vi "Highpass (Host).vi"() -> ()   [LabVIEW 2023]
uses:
  <vilib>/rvi/interface/nirviMethod/nirviMethod.xnode
  <vilib>/rvi/interface/nirviOpenFPGA/nirviOpenFPGA.xnode
  <vilib>/rvi/interface/nirviCloseFPGA/nirviCloseFPGA.xnode
  <vilib>/rvi/errors/niLvFpgaMergeErrorWithErrorCode.vi
  Highpass (FPGA).vi
  FPGA Bitfiles/highpass_FPGATarget_Highpass(FPGA)_je9PWvtYWXA.lvbitx
  <vilib>/userdefined/High Color/nirio_resource_hc.ctl
panel:
  in  "resource name":T1
  out "Filtered Signal":dbl[](graph)
  in  "stop":bool
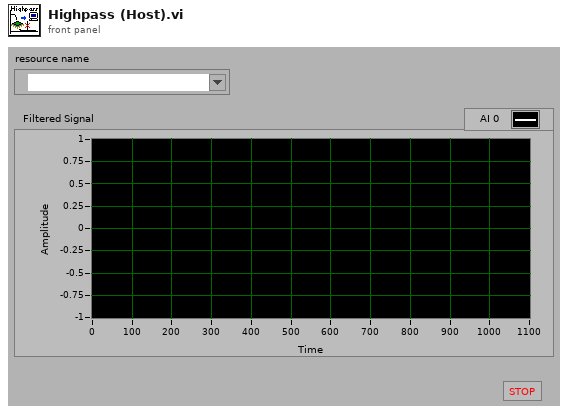
[diagram p1: front panel]
types:
  T1 = typedef "nirio_resource_hc.ctl" = tag
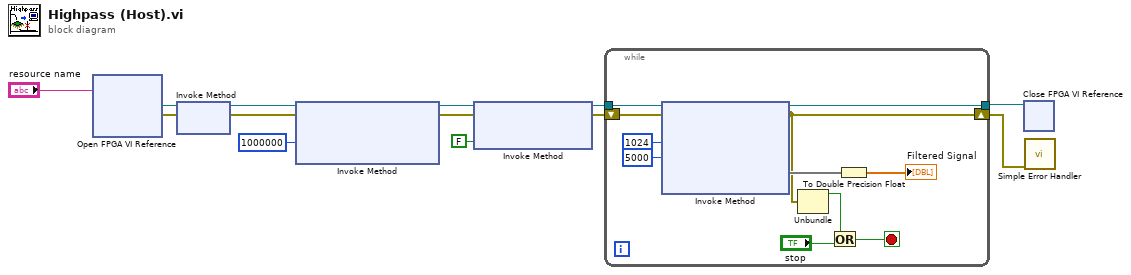
[diagram p0: block diagram]
diagram:
  n1 = xnode "Open FPGA VI Reference"("resource name"="resource name") -> ("FPGA VI Reference Out"=w13:refnum<k20>, "error out"=w12:errorcluster)  [unwired: 1 in]
  n2 = xnode "Invoke Method"("FPGA VI Reference In"=w13, "error in"=w12) -> ("FPGA VI Reference Out"=w10:refnum<k20>, "error out"=w11:errorcluster)
  n3 = xnode "Invoke Method"("FPGA VI Reference In"=w10, "error in"=w11, "Requested Depth"=u32 1000000 ("Depth")) -> ("FPGA VI Reference Out"=w7:refnum<k20>, "error out"=w8:errorcluster)  [unwired: 1 out]
  n4 = xnode "Invoke Method"("FPGA VI Reference In"=w7, "error in"=w8, "Wait Until Done (F)"=FALSE) -> ("FPGA VI Reference Out"=w4:refnum<k20>, "error out"=w5:errorcluster)
  n5 = while {
    tunnel: w4 -> [w24]
    shift-right: [w14] -> w3
    shift-left: w5 -> [w23]
    tunnel: [w16] -> w2
    stop <- w17 stop-if-true
    n6 = xnode "Invoke Method"("FPGA VI Reference In"=w24, "error in"=w23, "Number of Elements"=u32 1024, "Timeout (ms)"=5000) -> ("FPGA VI Reference Out"=w16:refnum<k20>, "error out"=w14:errorcluster, "Data"=w20:void[])  [unwired: 1 out]
    n7 = Unbundle(w14) -> ("status"=w18:bool)  [unwired: 2 out]
    n8 = Or(x=w18, y="stop") -> (x .or. y?=w17:bool)
    n9 = To Double Precision Float(number=w20) -> (double precision float=→"Filtered Signal":dbl[])
  }
  n10 = xnode "Close FPGA VI Reference"("FPGA VI Reference In"=w2) -> ()  [unwired: 1 in, 1 out]
  n11 = call <vilib>:"Simple Error Handler.vi"("error in (no error)"=w3) -> ()  [unwired: 1 in, 8 out]
